vi "Read datatype.vi"(8 "error in":errorcluster, 11 "VoidPointer in":refnum<class "VoidPointer.lvclass">) -> (0 "error out":errorcluster, 2 "datatype":string, 3 "VoidPointer out":refnum<class "VoidPointer.lvclass">)   [LabVIEW 2018, in "VoidPointer.lvclass"]
uses:
  VoidPointer.lvclass
  VoidPointer.lvclass/VoidPointer.ctl
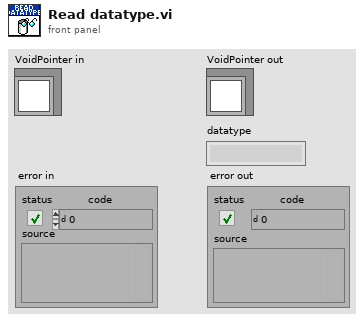
[diagram p1: front panel]
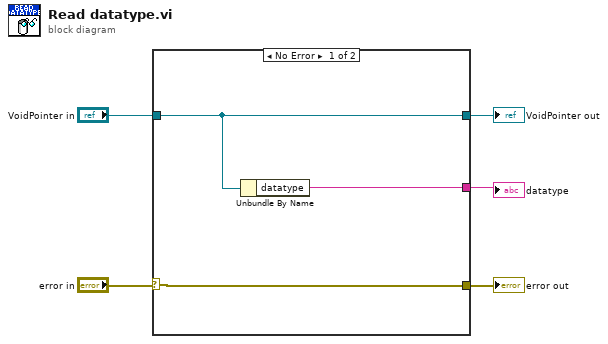
[diagram p0: block diagram]
diagram:
  n1 = case shown="No Error" "error in" {
    selector: "error in" -> [w8 w9]
    tunnel: [w8 w9] -> w4
    tunnel: [w7 w10] -> w3
    tunnel: "VoidPointer in" -> [w7 w10]
    tunnel: [w6 _] -> w1
    frame No Error {
      n2 = Unbundle By Name(w7) -> ("datatype"=w6:string)
    }
    frame Error {
    }
  }
  "error out" <- w4
  "VoidPointer out" <- w3
  "datatype" <- w1
